vi "Process_Create.vi"(5 "State":T6(ring)=enum."Standard", 7 "Activate?":bool, 8 "error in (no error)":errorcluster, 9 "Application Directory":path, 10 "Data in":T3, 11 "Name":string) -> (0 "error out":errorcluster, 3 "ref out":T2)   [LabVIEW 2015]
doc: "Use this template to build a VI to use as a subVI."
uses:
  Control/Process_Data.ctl
  Control/Process_Mode.ctl
  Control/Process_Function.ctl
  Control/Process_ref.ctl
  Control/Process_Flag.ctl
  0.GUI/Control/AllRef.ctl
panel:
  in  "Flag in":T1
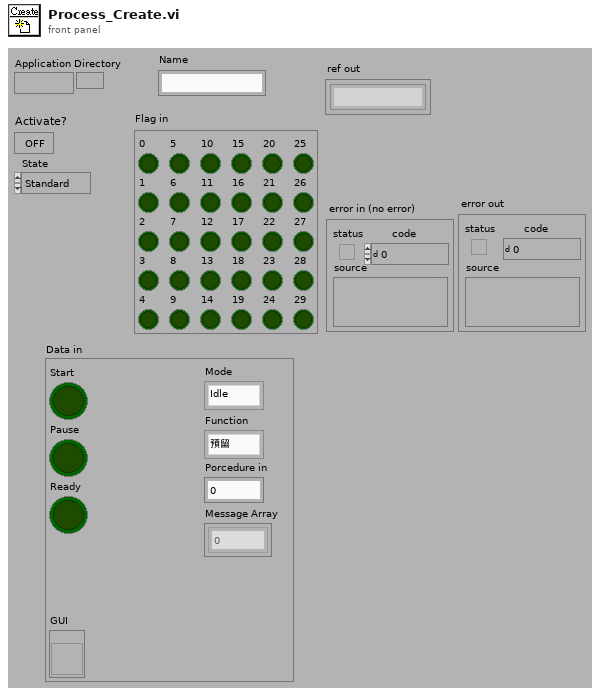
[diagram p1: front panel]
types:
  T1 = typedef "Process_Flag.ctl" = cluster{"0":bool, "1":bool, "2":bool, "3":bool, "4":bool, "5":bool, "6":bool, "7":bool, "8":bool, "9":bool, "10":bool, "11":bool, "12":bool, "13":bool, "14":bool, "15":bool, "16":bool, "17":bool, "18":bool, "19":bool, "20":bool, "21":bool, "22":bool, "23":bool, "24":bool, "25":bool, "26":bool, "27":bool, "28":bool, "29":bool}
  T2 = typedef "Process_ref.ctl" = refnum<k1>
  T3 = typedef "Process_Data.ctl" = cluster{"GUI":refnum<vi>, "Ready":bool, "Mode":T4, "Function":T5, "Porcedure in":u8, "Message Array":i32[], "Start":bool, "Pause":bool}
  T4 = typedef "Process_Mode.ctl" = enum8{"Idle", "Run", "Pause", "Err"}
  T5 = typedef "Process_Function.ctl" = enum8{"預留"}
  T6 = enum32{"Invalid", "Standard", "Closed", "Hidden", "Minimized", "Maximized"}
  T7 = typedef "AllRef.ctl" = cluster{"Error站ref":T8}
  T8 = typedef "Error站_ref.ctl" = refnum<k1>
  T9 = enum16{"OpenReference", "CloseReference", "Get Data", "Set Data", "Set Flag"}
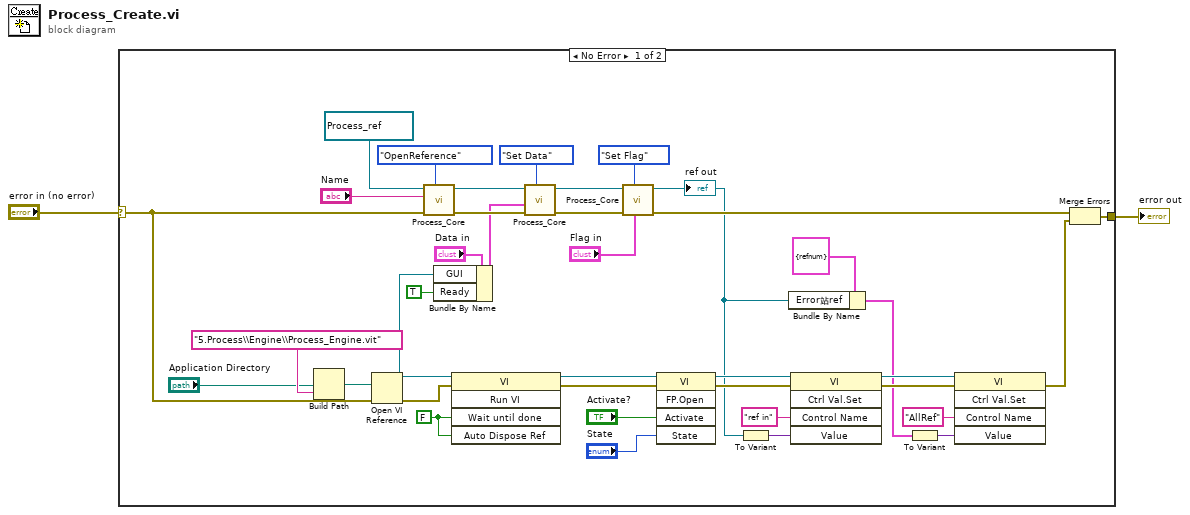
[diagram p0: block diagram]
diagram:
  n1 = case shown="No Error" "error in (no error)" {
    selector: "error in (no error)" -> [w12 w40]
    tunnel: [w37 w40] -> w1
    frame No Error {
      w11 = T2 refnum items=["Process_ref"] ("ref in")
      w33 = FALSE ("Wait until done")
      n2 = Build Path(base path="Application Directory", name or relative path="5.Process\\Engine\\Process_Engine.vit") -> (appended path=w23:path)
      n3 = Open VI Reference(vi path=w23, error in (no error)=w12) -> (vi reference=w14:refnum<vi>, error out=w34:errorcluster)  [unwired: 4 in]
      n4 = call "Process_Core.vi"("Function"=T9."OpenReference", "error in"=w12, "Name"="Name", "ref in"=w11) -> ("error out"=w39:errorcluster, "ref out"=w36:T2)  [unwired: 4 in, 2 out]
      n5 = Bundle By Name(cluster="Data in", "GUI"=w14, "Ready"=TRUE) -> (w21:T3)
      n6 = invoke class="VI" method="Run VI"(reference=w14, error in=w34, "Wait until done"=w33, "Auto Dispose Ref"=w33) -> (reference out=w31:refnum<vi>, error out=w32:errorcluster)  [unwired: 1 in, 3 out]
      n7 = call "Process_Core.vi"("Function"=T9."Set Data", "error in"=w39, "Data in"=w21, "ref in"=w36) -> ("error out"=w38:errorcluster, "ref out"=w20:T2)  [unwired: 4 in, 2 out]
      n8 = call "Process_Core.vi"("Flag in"="Flag in", "Function"=T9."Set Flag", "ref in"=w20) -> ("ref out"=w6:T2)  [unwired: 5 in, 3 out]
      "ref out" <- w6
      n9 = invoke class="VI" method="FP.Open"(reference=w31, error in=w32, "Activate"="Activate?", "State"="State") -> (reference out=w35:refnum<vi>, error out=w18:errorcluster)  [unwired: 1 in, 3 out]
      n10 = To Variant(anything=w6) -> (Variant=w15:variant)
      n11 = Bundle By Name(cluster=T7 {"Error站ref"=refnum} ("AllRef"), "Error站ref"=w6) -> (w3:T7)
      n12 = invoke class="VI" method="Ctrl Val.Set"(reference=w35, error in=w18, "Control Name"="ref in", "Value"=w15) -> (reference out=w8:refnum<vi>, error out=w9:errorcluster)  [unwired: 1 in, 3 out]
      n13 = To Variant(anything=w3) -> (Variant=w4:variant)
      n14 = invoke class="VI" method="Ctrl Val.Set"(reference=w8, error in=w9, "Control Name"="AllRef", "Value"=w4) -> (error out=w10:errorcluster)  [unwired: 1 in, 4 out]
      n15 = Merge Errors(w38, w10) -> (w37:errorcluster)
    }
    frame Error {
    }
  }
  "error out" <- w1
